vi "Read_Address_Map.vi"(8 "error in":errorcluster, 11 "file path":path=path "C:/Users/liyu/Desktop/flash map.xlsx") -> (0 "error out":errorcluster, 3 "all rows":string[][](array[string]))   [LabVIEW 2016]
uses:
  <vilib>/addons/_office/excel.llb/Excel Get Data ([str]).vi
  <vilib>/Utility/NIReport.llb/NI_report.lvclass
  <vilib>/addons/_office/NI_ReportGenerationToolkit.lvlib
  <vilib>/Utility/NIReport.llb/Excel/NI_Excel.lvclass
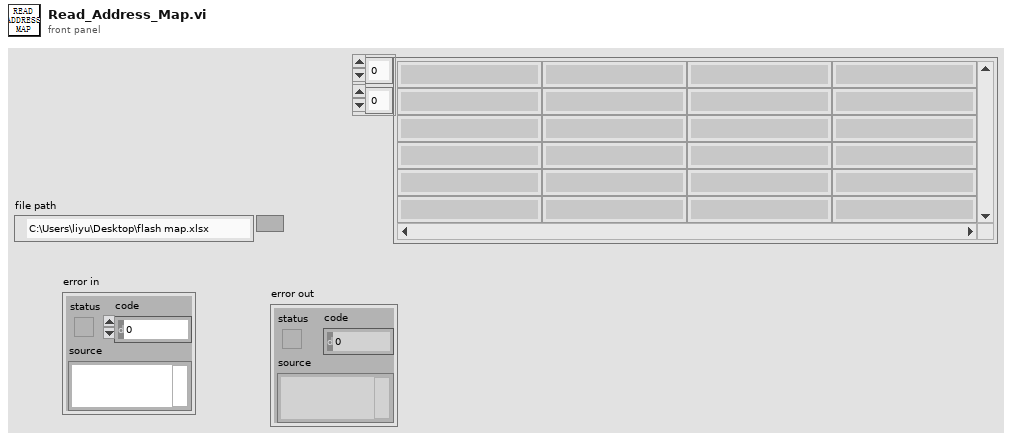
[diagram p1: front panel]
types:
  T1 = enum16{"Standard Report", "HTML", "Word", "Excel"}
  T2 = enum16{"maximized", "minimized", "normal", "no change"}
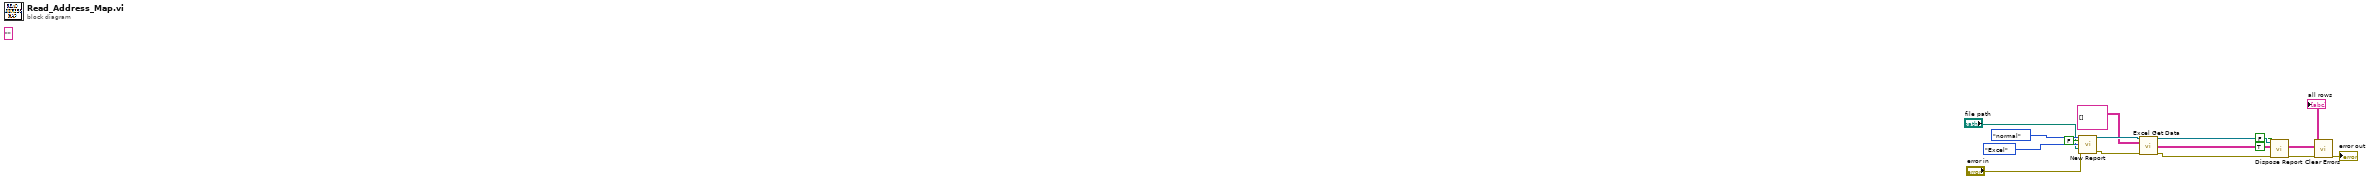
[diagram p0: block diagram]
diagram:
  (unwired) "" ("String")
  n1 = call <vilib>:"New Report.vi"("window state (normal)"=T2."normal", "display alerts? (F)"=FALSE, "report type"=T1."Excel", "template (empty)"="file path", "error in (no error)"="error in") -> ("report out"=w12:refnum<class "NI_report.lvclass">, "error out"=w11:errorcluster)  [unwired: 9 in]
  n2 = call-poly <vilib>:"Excel Get Data.vi"("report in"=w12, "data type"=string[][] [] ("all rows"), "error in (no error)"=w11) -> ("report out"=w7:refnum<class "NI_report.lvclass">, "data"=→"all rows":string[][], "error out"=w8:errorcluster)  [unwired: 10 in]
  n3 = call-dynamic "Dispose Report.vi"("report in"=w7, "wait until printing completed? (T)"=TRUE, "save changes? (F)"=FALSE, "error in (no error)"=w8) -> ("error out"=w4:errorcluster)  [unwired: 11 in]
  n4 = call <vilib>:"Clear Errors.vi"("error in (no error)"=w4) -> ("error out"=→"error out":errorcluster)  [unwired: 5 in, 1 out]
